vi "MRay Calculate Vision.vi"() -> ()   [LabVIEW 2011]
uses:
  <vilib>/vision/NI_Vision_Development_Module.lvlib
  Robot Global Data.vi
  <vilib>/Rock Robotics/WPI/Camera/WPI_CameraWhite Balance Values.ctl
panel:
  out "Turret Rotation":dbl
  in  "Pause":bool
  out "Target 4":dbl[](array[numeric])
  out "Target 3":dbl[](array[numeric])
  out "Target 2":dbl[](array[numeric])
  out "Target 1":dbl[](array[numeric])
  in  "Turret Speed Limit":dbl=0.3
  out "Number of Rectangles Visible":dbl
  out "Y Position Array":dbl[](array[numeric])
  out "X Position Array":dbl[](array[numeric])
  out "Processed Image":T1(plugin-control)
  out "Original Image":T1(plugin-control)
  in  "Annotate":bool=TRUE
  in  "Particle Count Limit":i32=10
  in  "Area Size Limit":i32=444
  in  "Range":cluster{"Lower value":sgl, "Upper value":sgl}={"Lower value"=120.0, "Upper value"=255.0}
  # "X Coord\nY Coord\nDistance"
  # "Light Intensity"
  # "-1 to 1"
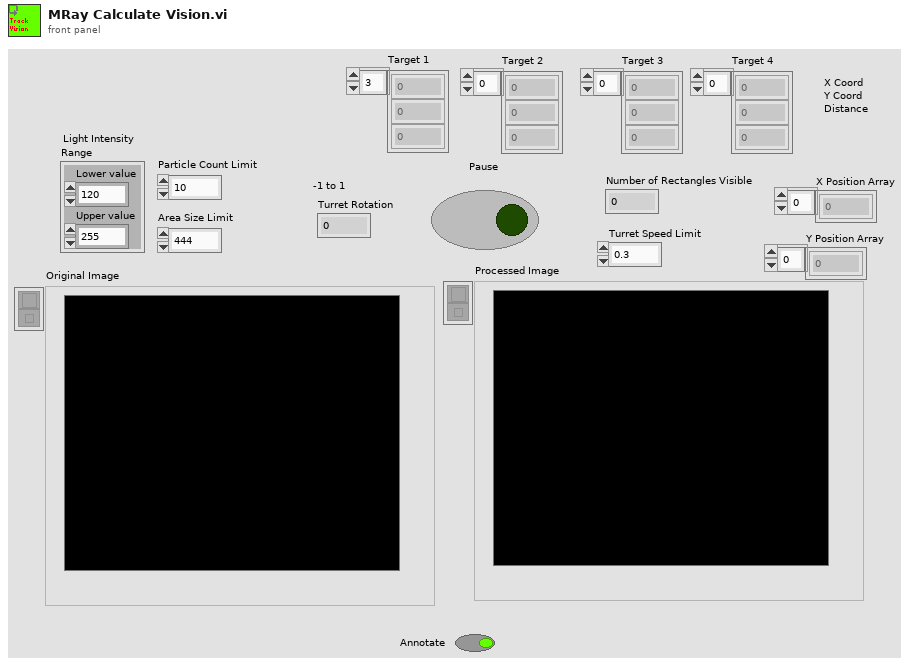
[diagram p1: front panel]
types:
  T1 = typedef "IMAQ Image.ctl" = refnum<image>
  T2 = typedef "WPI_CameraWhite Balance Values.ctl" = enum16{"Auto", "Fixed indoor", "Fixed outdoor 1", "Fixed outdoor 2", "Fixed fluorescent 1", "Fixed fluorescent 2", "Hold current"}
  T3 = cluster{"Rect Coverage":dbl, "Aspect Ratio":dbl, "X Edge Strength":dbl, "Y Edge Strength":dbl}
  T4 = cluster{"Position":cluster{"X":dbl, "Y":dbl}, "Distance (ft)":dbl}[]
  T5 = typedef "Image Type" = u32
  T6 = typedef "WPI_CameraImageSize.ctl" = enum16{"640x480", "320x240", "160x120"}
  T7 = cluster{"fps":i32, "compression":i32, "Image Size":T6}
  T8 = typedef "WPI_CameraDevRef.ctl" = cluster{"Camera Address":string, "CameraStatus":errorcluster, "Acquire Image Notifier":refnum<notifier>}
  T9 = cluster{cluster{"Left":dbl, "Top":dbl, "Right":dbl, "Bottom":dbl}, dbl[]}[]
  T10 = cluster{"Left":dbl, "Top":dbl, "Right":dbl, "Bottom":dbl}
  T11 = cluster{"Target Center (-1 to 1)":cluster{"X":dbl, "Y":dbl}, "Distance (ft)":dbl}
  T12 = cluster{"Target Center (-1 to 1)":cluster{"X":dbl, "Y":dbl}, "Distance (ft)":dbl}[]
  T13 = cluster{"Position":cluster{"X":dbl, "Y":dbl}, "Distance (ft)":dbl}
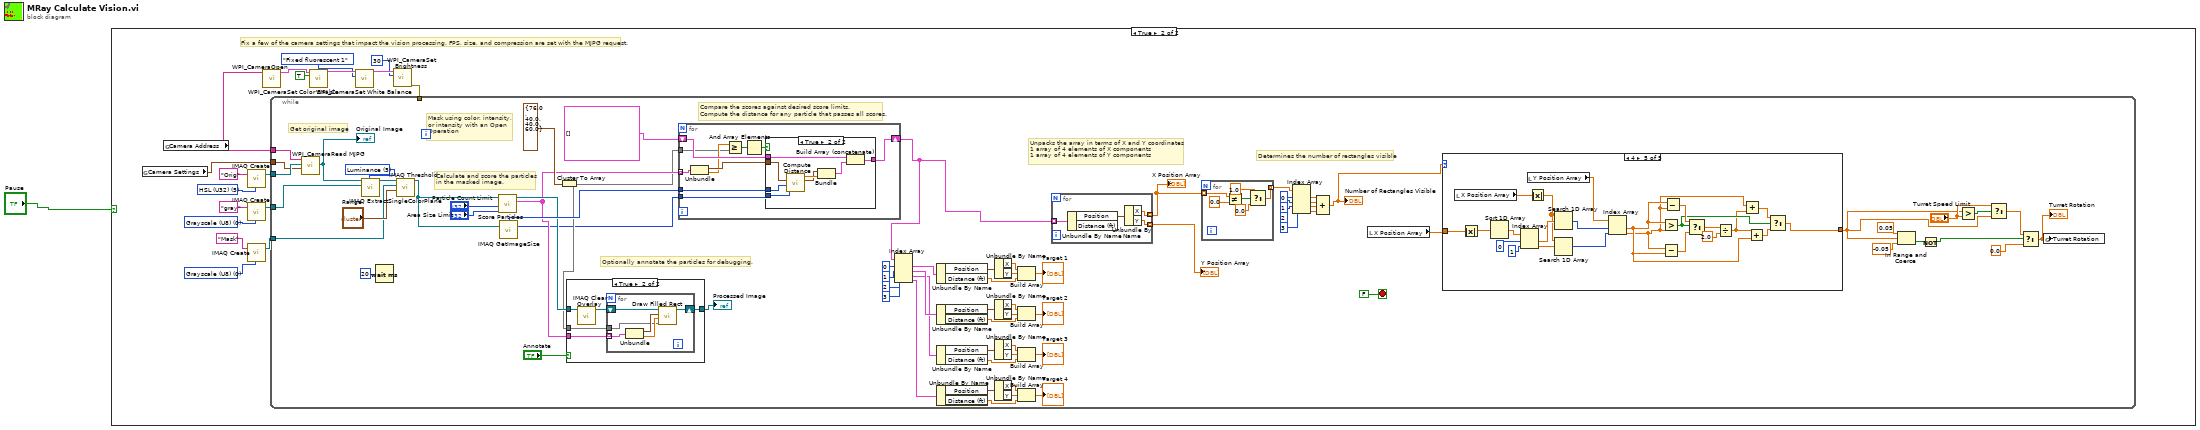
[diagram p0: block diagram]
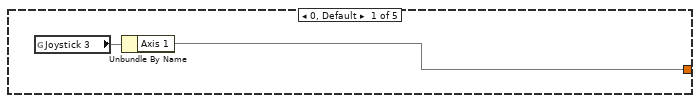
[diagram p3: hidden frame]
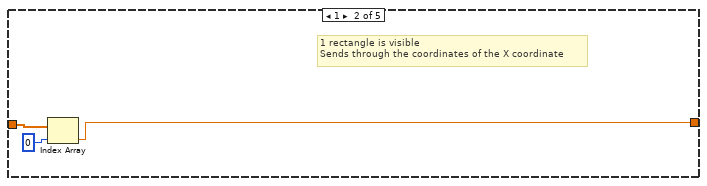
[diagram p4: hidden frame]
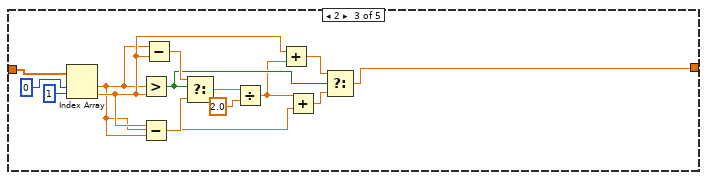
[diagram p5: hidden frame]
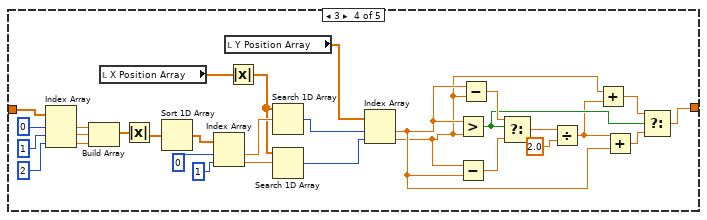
[diagram p6: hidden frame]
diagram:
  n1 = case shown="True" "Pause" {
    frame False {
    }
    frame True {
      w12 = T5 0 items=["Grayscale (U8)", "Grayscale (I16)", "Grayscale (SGL)", "Complex (CSG)", "RGB (U32)", "HSL (U32)", "RGB (U64)", "Grayscale (U16)"] ("Image Type")
      w16 = T5 5 items=["Grayscale (U8)", "Grayscale (I16)", "Grayscale (SGL)", "Complex (CSG)", "RGB (U32)", "HSL (U32)", "RGB (U64)", "Grayscale (U16)"] ("Image Type")
      w19 = T5 0 items=["Grayscale (U8)", "Grayscale (I16)", "Grayscale (SGL)", "Complex (CSG)", "RGB (U32)", "HSL (U32)", "RGB (U64)", "Grayscale (U16)"] ("Image Type")
      # "Fix a few of the camera settings that impact the vision processing. FPS, size, and compression are set with the MJPG request."
      n2 = global read "Robot Global Data.vi" "Camera Settings"() -> (w2:T7)
      n3 = global read "Robot Global Data.vi" "Camera Address"() -> (w3:string)
      n4 = call "IMAQ Create"("Image Name"="Orig", "Image Type"=w16) -> ("New Image"=w15:T1)  [unwired: 2 in, 2 out]
      n5 = call "IMAQ Create"("Image Name"="gray", "Image Type"=w19) -> ("New Image"=w14:T1)  [unwired: 2 in, 2 out]
      n6 = call "IMAQ Create"("Image Name"="Mask", "Image Type"=w12) -> ("New Image"=w11:T1)  [unwired: 2 in, 2 out]
      n7 = call <vilib>:"WPI_CameraOpen.vi"("Camera Address"=w3) -> ("CameraDevRef"=w10:T8)  [unwired: 9 in, 1 out]
      n8 = call <vilib>:"WPI_CameraSet Color Enable.vi"("Color Enabled"=TRUE, "CameraDevRef"=w10) -> ("CameraDevRef Out"=w8:T8)  [unwired: 8 in, 1 out]
      n9 = call <vilib>:"WPI_CameraSet White Balance.vi"("White Balance"=WPI_CameraWhite_Balance_Values."Fixed fluorescent 1", "CameraDevRef"=w8) -> ("CameraDevRef Out"=w6:T8)  [unwired: 8 in, 1 out]
      n10 = call <vilib>:"WPI_CameraSet Brightness.vi"("Brightness"=30, "CameraDevRef"=w6) -> ("error out"=w4:errorcluster)  [unwired: 8 in, 1 out]
      n11 = while {
        tunnel: w15 -> [w93]
        tunnel: w14 -> [w75]
        tunnel: w11 -> [w77]
        tunnel: w3 -> [w92]
        tunnel: w4 -> [_]
        tunnel: w2 -> [w81]
        stop <- FALSE stop-if-true
        w80 = 5 items=["Red", "Green", "Blue", "Hue", "Saturation", "Luminance", "Value", "Intensity"] ("Color Plane")
        # "Determines the number of rectangles visible"
        # "Unpacks the array in terms of X and Y coordinates\n1 array of 4 elements of X components\n1 array of 4 elements of Y components"
        # "Optionally annotate the particles for debugging."
        # "Compare the scores against desired score limits.\nCompute the distance for any particle that passes all scores."
        # "Calculate and score the particles\nin the masked image."
        # "Mask using color, intensity,\nor intensity with an Open\nOperation"
        # "Get original image"
        n12 = call <vilib>:"WPI_CameraRead MJPG.vi"("Camera Settings"=w81, "Image"=w93, "address"=w92) -> ("Image Out"=w76:T1)  [unwired: 7 in, 1 out]
        "Original Image" <- w76
        n13 = call "IMAQ ExtractSingleColorPlane"("Color Plane"=w80, "Image Dst"=w75, "Image Src"=w76) -> ("Image Dst Out"=w78:T1)  [unwired: 1 in, 7 out]
        n14 = Wait (ms)(milliseconds to wait=u32 20) -> ()  [unwired: 1 out]
        n15 = call "IMAQ Threshold"("Range"="Range", "Image Dst"=w77, "Image Src"=w78) -> ("Image Dst Out"=w74:T1)  [unwired: 3 in, 5 out]
        n16 = call "Score Particles.vi"("Area Size Limit"="Area Size Limit", "Particle Count Limit"="Particle Count Limit", "Image Refnum in"=w74) -> ("Scored Particle Info"=w88:T9, "Image Refnum out"=w91:T1)  [unwired: 6 in, 1 out]
        n17 = call "IMAQ GetImageSize"("Image"=w74) -> ("Y Resolution"=w82:i32, "X Resolution"=w94:i32)  [unwired: 3 in, 1 out]
        n18 = Cluster To Array(cluster=T3 {"Rect Coverage"=76.0, "Aspect Ratio"=40.0, "X Edge Strength"=40.0, "Y Edge Strength"=60.0} ("Score Limits")) -> (array=w86:dbl[])
        n19 = case shown="True" "Annotate" {
          tunnel: w91 -> [w177 w182]
          tunnel: [w177 w181] -> w89
          tunnel: w88 -> [_ w179]
          tunnel: w86 -> [_ w178]
          frame False {
          }
          frame True {
            n20 = call "IMAQ Clear Overlay"("Image"=w182) -> ("Image Out"=w180:T1)  [unwired: 2 in, 8 out]
            n21 = for {
              shift-right: [w187] -> w181
              shift-left: w180 -> [w188]
              tunnel: w179 -> [w184] mode=indexing
              tunnel: w178 -> [w183]
              n22 = Unbundle(w184) -> (w185:T10, w186:dbl[])
              n23 = call "Draw Filled Rect.vi"("Limits"=w183, "Scores"=w186, "Bounding Box"=w185, "image in"=w188) -> ("image out"=w187:T1)  [unwired: 7 in]
            }
          }
        }
        "Processed Image" <- w89
        n24 = for {
          shift-right: [w197] -> w46
          shift-left: T4 [] -> [w198]
          tunnel: w94 -> [w196]
          tunnel: w88 -> [w194] mode=indexing
          tunnel: w86 -> [w190]
          tunnel: w82 -> [w189]
          n25 = Unbundle(w194) -> (w195:T10, w191:dbl[])
          n26 = Greater Or Equal?(x=w191, y=w190) -> (x >= y?=w193:bool[])
          n27 = And Array Elements(Boolean array=w193) -> (logical AND=w192:bool)
          n28 = case shown="True" w192 {
            tunnel: w198 -> [w199 w207]
            tunnel: [w199 w206] -> w197
            tunnel: w195 -> [_ w202]
            tunnel: w196 -> [_ w204]
            tunnel: w189 -> [_ w200]
            frame False {
            }
            frame True {
              n29 = call "Compute Distance.vi"("Y Image Resolution"=w200, "X Image Resolution"=w204, "Bounding Box"=w202) -> ("Target Center (-1 to 1)"=w201:cluster{"X":dbl, "Y":dbl}, "Distance (ft)"=w203:dbl)  [unwired: 7 in]
              n30 = Bundle("Target Center (-1 to 1)"=w201, "Distance (ft)"=w203) -> (w205:T11)  [unwired: 1 in]
              n31 = Build Array (concatenate)(w207, w205) -> (w206:T12)
            }
          }
        }
        n32 = Index Array(array=w46, index #1=0 ("index"), index #2=1 ("index"), index #3=2 ("index"), index #4=3 ("index")) -> (element #1=w43:T13, element #2=w34:T13, element #3=w28:T13, element #4=w20:T13)
        n33 = Unbundle By Name(w43) -> ("Position"=w42:cluster{"X":dbl, "Y":dbl}, "Distance (ft)"=w39:dbl)
        n34 = Unbundle By Name(w34) -> ("Position"=w35:cluster{"X":dbl, "Y":dbl}, "Distance (ft)"=w37:dbl)
        n35 = Unbundle By Name(w28) -> ("Position"=w31:cluster{"X":dbl, "Y":dbl}, "Distance (ft)"=w29:dbl)
        n36 = Unbundle By Name(w20) -> ("Position"=w23:cluster{"X":dbl, "Y":dbl}, "Distance (ft)"=w25:dbl)
        n37 = Unbundle By Name(w42) -> ("X"=w41:dbl, "Y"=w40:dbl)
        n38 = Unbundle By Name(w35) -> ("X"=w33:dbl, "Y"=w36:dbl)
        n39 = Unbundle By Name(w31) -> ("X"=w27:dbl, "Y"=w30:dbl)
        n40 = Unbundle By Name(w23) -> ("X"=w21:dbl, "Y"=w24:dbl)
        n41 = Build Array(w41, w40, w39) -> (→"Target 1":dbl[])
        n42 = Build Array(w33, w36, w37) -> (→"Target 2":dbl[])
        n43 = Build Array(w27, w30, w29) -> (→"Target 3":dbl[])
        n44 = Build Array(w21, w24, w25) -> (→"Target 4":dbl[])
        n45 = for {
          tunnel: [w175] -> w44 mode=indexing
          tunnel: [w174] -> w62 mode=indexing
          tunnel: w46 -> [w173] mode=indexing
          n46 = Unbundle By Name(w173) -> ("Position"=w176:cluster{"X":dbl, "Y":dbl})  [unwired: 1 out]
          n47 = Unbundle By Name(w176) -> ("X"=w174:dbl, "Y"=w175:dbl)
        }
        "X Position Array" <- w62
        "Y Position Array" <- w44
        n48 = for {
          tunnel: w62 -> [w99] mode=indexing
          tunnel: [w95] -> w61 mode=indexing
          n49 = Not Equal?(x=w99, y=0.0) -> (x != y?=w98:bool)
          n50 = Select(t=1.0, s=w98, f=0.0) -> (s? t:f=w95:dbl)
        }
        n51 = Index Array(array=w61, index #1=0 ("index"), index #2=1 ("index"), index #3=2 ("index"), index #4=3 ("index")) -> (element #1=w59:dbl, element #2=w60:dbl, element #3=w58:dbl, element #4=w57:dbl)
        n52 = Compound Arithmetic op=ADD(w59, w60, w58, w57) -> (w51:dbl)
        "Number of Rectangles Visible" <- w51
        n53 = local read "X Position Array"() -> (w72:dbl[])
        n54 = case shown="4" w51 {
          tunnel: w72 -> [_ w105 w119 w149 w152]
          tunnel: [w101 w103 w106 w121 w151] -> w63
          frame 0, Default {
            n55 = global read "Robot Global Data.vi" "Joystick 3"() -> (w102)
            n56 = Unbundle By Name(w102) -> ("Axis 1"=w101)
          }
          frame 1 {
            # "1 rectangle is visible\nSends through the coordinates of the X coordinate"
            n57 = Index Array(array=w105, index=0) -> (element=w103:dbl)
          }
          frame 2 {
            n58 = Index Array(array=w119, index #1=0 ("index"), index #2=1 ("index")) -> (element #1=w107:dbl, element #2=w108:dbl)
            n59 = Greater?(x=w107, y=w108) -> (0:w112:bool)
            n60 = Subtract(x=w108, y=w107) -> (x-y=w115:dbl)
            n61 = Subtract(x=w107, y=w108) -> (x-y=w116:dbl)
            n62 = Select(t=w116, s=w112, f=w115) -> (s? t:f=w114:dbl)
            n63 = Divide(x=w114, y=2.0) -> (x/y=w109:dbl)
            n64 = Add(x=w108, y=w109) -> (x+y=w111:dbl)
            n65 = Add(x=w109, y=w107) -> (x+y=w110:dbl)
            n66 = Select(t=w111, s=w112, f=w110) -> (s? t:f=w106:dbl)
          }
          frame 3 {
            n67 = Index Array(array=w149, index #1=0 ("index"), index #2=1 ("index"), index #3=2 ("index")) -> (element #1=w145:dbl, element #2=w144:dbl, element #3=w143:dbl)
            n68 = Build Array(w145, w144, w143) -> (w142:dbl[])
            n69 = local read "X Position Array"() -> (w135:dbl[])
            n70 = Absolute Value(x=w142) -> (abs(x)=w141:dbl[])
            n71 = Sort 1D Array(array=w141) -> (sorted array=w140:dbl[])
            n72 = Index Array(array=w140, index #1=0 ("index"), index #2=1 ("index")) -> (element #1=w137:dbl, element #2=w136:dbl)
            n73 = local read "Y Position Array"() -> (w133:dbl[])
            n74 = Absolute Value(x=w135) -> (abs(x)=w120:dbl[])
            n75 = Search 1D Array(1D array=w120, element=w137) -> (index of element=w134:i32)  [unwired: 1 in]
            n76 = Search 1D Array(1D array=w120, element=w136) -> (index of element=w132:i32)  [unwired: 1 in]
            n77 = Index Array(array=w133, index #1=w134, index #2=w132) -> (element #1=w123:dbl, element #2=w122:dbl)
            n78 = Greater?(x=w123, y=w122) -> (0:w127:bool)
            n79 = Subtract(x=w122, y=w123) -> (x-y=w130:dbl)
            n80 = Subtract(x=w123, y=w122) -> (x-y=w131:dbl)
            n81 = Select(t=w131, s=w127, f=w130) -> (s? t:f=w129:dbl)
            n82 = Divide(x=w129, y=2.0) -> (x/y=w124:dbl)
            n83 = Add(x=w122, y=w124) -> (x+y=w126:dbl)
            n84 = Add(x=w124, y=w123) -> (x+y=w125:dbl)
            n85 = Select(t=w126, s=w127, f=w125) -> (s? t:f=w121:dbl)
          }
          frame 4 {
            n86 = local read "X Position Array"() -> (w166:dbl[])
            n87 = Absolute Value(x=w152) -> (abs(x)=w172:dbl[])
            n88 = Sort 1D Array(array=w172) -> (sorted array=w171:dbl[])
            n89 = Index Array(array=w171, index #1=0 ("index"), index #2=1 ("index")) -> (element #1=w168:dbl, element #2=w167:dbl)
            n90 = local read "Y Position Array"() -> (w164:dbl[])
            n91 = Absolute Value(x=w166) -> (abs(x)=w150:dbl[])
            n92 = Search 1D Array(1D array=w150, element=w168) -> (index of element=w165:i32)  [unwired: 1 in]
            n93 = Search 1D Array(1D array=w150, element=w167) -> (index of element=w163:i32)  [unwired: 1 in]
            n94 = Index Array(array=w164, index #1=w165, index #2=w163) -> (element #1=w154:dbl, element #2=w153:dbl)
            n95 = Greater?(x=w154, y=w153) -> (0:w158:bool)
            n96 = Subtract(x=w153, y=w154) -> (x-y=w161:dbl)
            n97 = Subtract(x=w154, y=w153) -> (x-y=w162:dbl)
            n98 = Select(t=w162, s=w158, f=w161) -> (s? t:f=w160:dbl)
            n99 = Divide(x=w160, y=2.0) -> (x/y=w155:dbl)
            n100 = Add(x=w153, y=w155) -> (x+y=w157:dbl)
            n101 = Add(x=w155, y=w154) -> (x+y=w156:dbl)
            n102 = Select(t=w157, s=w158, f=w156) -> (s? t:f=w151:dbl)
          }
        }
        n103 = In Range and Coerce(upper limit=0.05, x=w63, lower limit=-0.05) -> (In Range?=w66:bool)  [unwired: 1 out]
        n104 = Not(x=w66) -> (.not. x?=w67:bool)
        n105 = Greater?(x=w63, y="Turret Speed Limit") -> (0:w69:bool)
        n106 = Select(t="Turret Speed Limit", s=w69, f=w63) -> (s? t:f=w71:dbl)
        n107 = Select(t=w71, s=w67, f=0.0) -> (s? t:f=w45:dbl)
        "Turret Rotation" <- w45
        n108 = global write "Robot Global Data.vi" "Turret Rotation"(w45) -> ()
      }
    }
  }
